vi "MathFunction.vi"(8 "error in (no error)":errorcluster, 9 "y":dbl, 10 "x":dbl, 11 "Add in":refnum<class "Subtract.lvclass">) -> (0 "error out":errorcluster, 2 "f(x,y)":dbl, 3 "Add out":refnum<class "Subtract.lvclass">)   [LabVIEW 2019, in "lv-classprovidershell-example.lvlib" / "Subtract.lvclass"]
uses:
  Subtract.lvclass
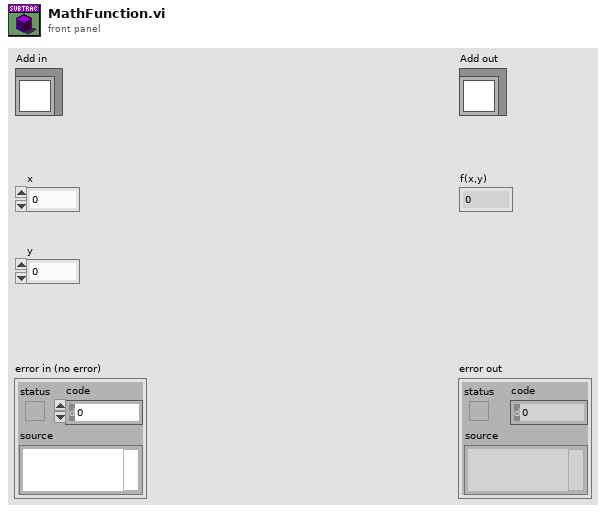
[diagram p1: front panel]
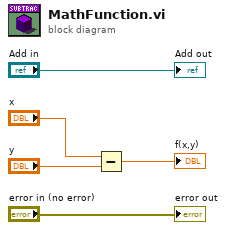
[diagram p0: block diagram]
diagram:
  n1 = Subtract(x="x", y="y") -> (x-y=→"f(x,y)":dbl)
  "error out" <- "error in (no error)"
  "Add out" <- "Add in"
